vi "AerotechHardwareAcquire.vi"(8 "error in (no error)":errorcluster, 11 "AerotechStage in":refnum<class "AerotechStage.lvclass">) -> (0 "error out":errorcluster, 3 "AerotechStage out":refnum<class "AerotechStage.lvclass">)   [LabVIEW 2020, in "AerotechStage.lvclass"]
uses:
  AerotechStage.lvclass
  Aerotech Acq FGV Control.ctl
  Aerotech Acq FGV Function.ctl
  AerotechStage.lvclass/AerotechStage.ctl
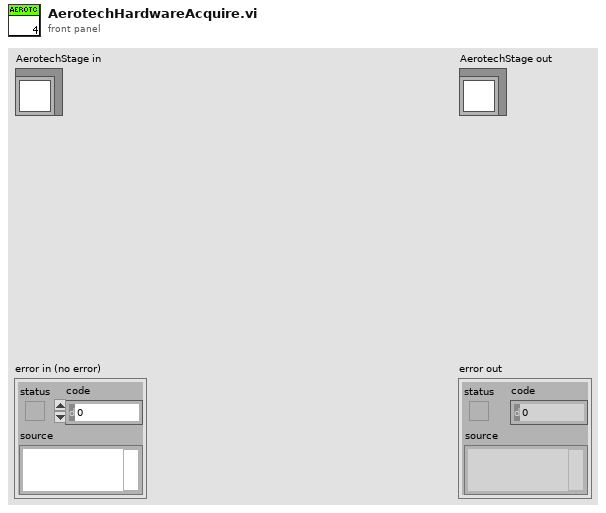
[diagram p1: front panel]
types:
  T1 = typedef "Aerotech Acq FGV Function.ctl" = enum16{"Clear", "Write", "Read"}
  T2 = typedef "Aerotech Acq FGV Control.ctl" = cluster{"Position":dbl[], "Power Status":bool[], "Move Active Status":bool[], "Busy Status":bool}
  T3 = typedef "ControllerDiagPacket.ctl" = cluster{"Count":i32, "Packet Time":i64, "Axes":T4[], "error":errorcluster}
  T4 = typedef "AxisDiagPacket.ctl" = cluster{"Axis Name":string, "Acceleration Command":dbl, "Amplifier Temperature":sgl, "Analog Input 0":dbl, "Analog Input 1":dbl, "Analog Output 0":dbl, "Analog Output 1":dbl, "Axis Fault (num)":i32, "Axis Fault (str)":string, "Axis Fault (bits)":cluster{"AmplifierFault":bool, "AmplifierTemperatureFault":bool, "CcwEndOfTravelLimitFault":bool, "CcwSoftwareLimitFault":bool, "CommunicationLostFault":bool, "CwEndOfTravelLimitFault":bool, "CwSoftwareLimitFault":bool, "EmergencyStopFault":bool, "EncoderFault":bool, "ExternalFault":bool, "FeedbackScalingFault":bool, "HallSensorFault":bool, "MarkerSearchFault":bool, "MaxVelocityCommandFault":bool, "MotorTemperatureFault":bool, "None":bool, "OverCurrentFault":bool, "PositionErrorFault":bool, "PositionFeedbackFault":bool, "PowerSupplyFault":bool, "VelocityErrorFault":bool, "VelocityFeedbackFault":bool, "VoltageClampFault":bool}, "Axis Status (num)":i32, "Axis Status (str)":string, "Axis Status (bits)":cluster{"AccelerationPhase":bool, "AutofocusActive":bool, "BrakeOutput":bool, "CalibrationActive":bool, "CalibrationEnabled":bool, "CcwEndOfTravelLimitInput":bool, "CommandShapingFilterDone":bool, "CosineEncoderError":bool, "CurrentClamp":bool, "CwEndOfTravelLimitInput":bool, "DecelerationPhase":bool, "EmergencyStopInput":bool, "Enabled":bool, "GantryMasterActive":bool, "GantryModeActive":bool, "HallAInput":bool, "HallBInput":bool, "HallCInput":bool, "Homed":bool, "HomeLimitInput":bool, "Homing":bool, "InPosition":bool, "InPosition2":bool, "JoystickControl":bool, "MarkerInput":bool, "MasterMotionSuppressed":bool, "MasterSlaveControl":bool, "MotionIsCw":bool, "MoveActive":bool, "None":bool, "PositionCaptureActive":bool, "ServoControl":bool, "SineEncoderError":bool}, "Current Command":sgl, "Current Error":sgl, "Current Feedback":sgl, "Digital Input 0":i32, "Digital Input 1":i32, "Digital Input 2":i32, "Digital Output 0":i32, "Digital Output 1":i32, "Digital Output 2":i32, "Position Feedback Auxiliary":dbl, "Position Command":dbl, "Position Error":dbl, "Position Feedback":dbl, "Program Position Command":dbl, "Program Position Error":dbl, "Program Position Feedback":dbl, "Velocity Command":dbl, "Velocity Error":dbl, "Velocity Feedback":dbl}
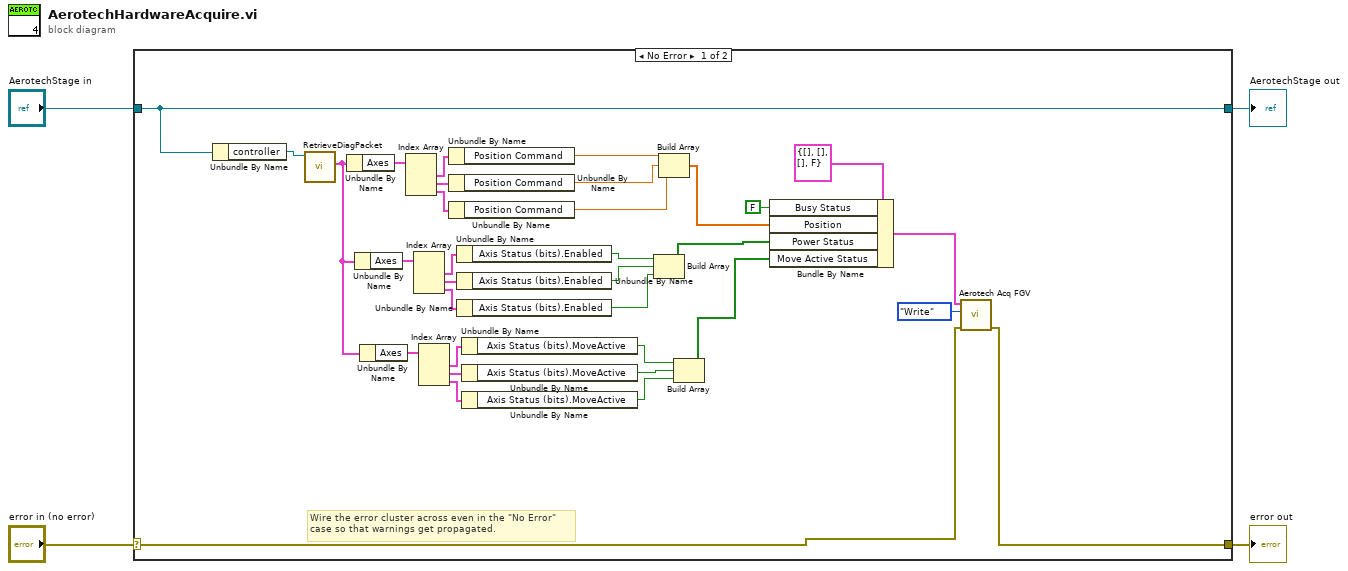
[diagram p0: block diagram]
diagram:
  n1 = case shown="No Error" "error in (no error)" {
    selector: "error in (no error)" -> [w6 w39]
    tunnel: [w5 w39] -> w3
    tunnel: [w37 w38] -> w1
    tunnel: "AerotechStage in" -> [w37 w38]
    frame No Error {
      # "Wire the error cluster across even in the \"No Error\"\ncase so that warnings get propagated."
      n2 = Unbundle By Name(w37) -> ("controller"=w36:refnum<k24>)
      n3 = call "RetrieveDiagPacket.vi"("Controller In"=w36) -> ("ControllerDiagPacket"=w27:T3)  [unwired: 8 in, 2 out]
      n4 = Unbundle By Name(w27) -> ("Axes"=w35:T4[])
      n5 = Unbundle By Name(w27) -> ("Axes"=w30:T4[])
      n6 = Unbundle By Name(w27) -> ("Axes"=w29:T4[])
      n7 = Index Array(array=w35) -> (element #1=w34:T4, element #2=w32:T4, element #3=w33:T4)  [unwired: 3 in]
      n8 = Index Array(array=w30) -> (element #1=w31:T4, element #2=w26:T4, element #3=w25:T4)  [unwired: 3 in]
      n9 = Index Array(array=w29) -> (element #1=w28:T4, element #2=w23:T4, element #3=w24:T4)  [unwired: 3 in]
      n10 = Unbundle By Name(w34) -> ("Position Command"=w22:dbl)
      n11 = Unbundle By Name(w32) -> ("Position Command"=w21:dbl)
      n12 = Unbundle By Name(w33) -> ("Position Command"=w20:dbl)
      n13 = Unbundle By Name(w31) -> ("Axis Status (bits).Enabled"=w19:bool)
      n14 = Unbundle By Name(w26) -> ("Axis Status (bits).Enabled"=w18:bool)
      n15 = Unbundle By Name(w25) -> ("Axis Status (bits).Enabled"=w17:bool)
      n16 = Unbundle By Name(w28) -> ("Axis Status (bits).MoveActive"=w16:bool)
      n17 = Unbundle By Name(w23) -> ("Axis Status (bits).MoveActive"=w15:bool)
      n18 = Unbundle By Name(w24) -> ("Axis Status (bits).MoveActive"=w14:bool)
      n19 = Build Array(w19, w18, w17) -> (w8:bool[])
      n20 = Build Array(w22, w21, w20) -> (w9:dbl[])
      n21 = Build Array(w16, w15, w14) -> (w7:bool[])
      n22 = Bundle By Name(cluster=T2 {"Position"=[], "Power Status"=[], "Move Active Status"=[], "Busy Status"=FALSE} ("Aerotech Acq Data"), "Busy Status"=FALSE, "Position"=w9, "Power Status"=w8, "Move Active Status"=w7) -> (w12:T2)
      n23 = call "Aerotech Acq FGV.vi"("error in (no error)"=w6, "Function"=Aerotech_Acq_FGV_Function."Write", "Aerotech Acq Data"=w12) -> ("error out"=w5:errorcluster)  [unwired: 7 in, 1 out]
    }
    frame Error {
    }
  }
  "error out" <- w3
  "AerotechStage out" <- w1
